vi "encoderValues.vi"() -> ()   [LabVIEW 2016]
panel:
  in  "Reset?":bool
  out "Right":dbl
  out "Left":dbl
  in  "prev. Right":dbl
  in  "prev. Left":dbl
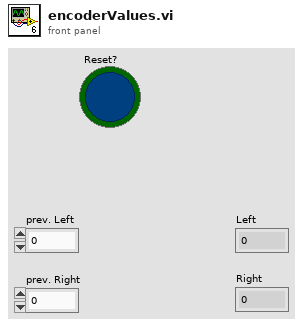
[diagram p1: front panel]
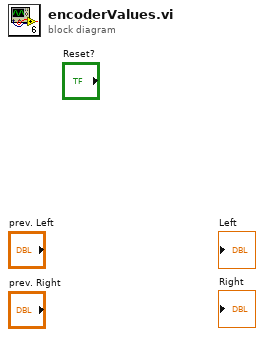
[diagram p0: block diagram]
diagram:
